vi "参数设置.vi"() -> ()   [LabVIEW 2018]
uses:
  globalMessage.vi
panel:
  in  "能量计量程":enum16{"200uJ", "20uJ", "2uJ", "200nJ"}(ring)
  in  "能量计通道":enum16{"Channel 1", "Channel 2"}(ring)=enum."Channel 2"
  in  "功率计通道":enum16{"Channel 1", "Channel 2"}(ring)
  in  "测量表头IP":string="192.168.129.77"
  in  "曝光时间 2":u64
  in  "模拟增益 2":u64
  in  "相机IP 2":string="192.168.1.10"
  in  "曝光时间":u64
  in  "模拟增益":u64
  in  "相机IP":string="192.168.1.10"
  in  "触发电压":u64(ring)=200 items=["200mv"=200, "20mv"=20, "2mv"=2]
  in  "时间范围":u64(ring)=100000 items=["100ms"=1000000000, "10ms"=100000000, "1ms"=10000000, "100us"=1000000, "10us"=100000, "1us"=10000, "100ns"=1000, "10ns"=100, "1ns"=10, "100ps"=1]
  in  "电压范围":u64(ring)=10 items=["1 V"=1000000, "100mv"=100000, "10mv"=10000, "1mv"=1000, "100uv"=100, "10uv"=10]
  in  "示波器通道":T1(ring)
  in  "工作波长（nm）":u32=400 min=400 max=1100
  in  "编号":string
  in  "激光器型号":string
  in  "确定":bool
  out "提示":string
  in  "error in (no error)":errorcluster
  # "通用参数"
  # "近场相机\n参数"
  # "远场相机\n参数"
  # "功率/能量计\n参数"
  # "示波器\n参数"
  # "偏振测量仪\n参数"
  # "光谱仪\n参数"
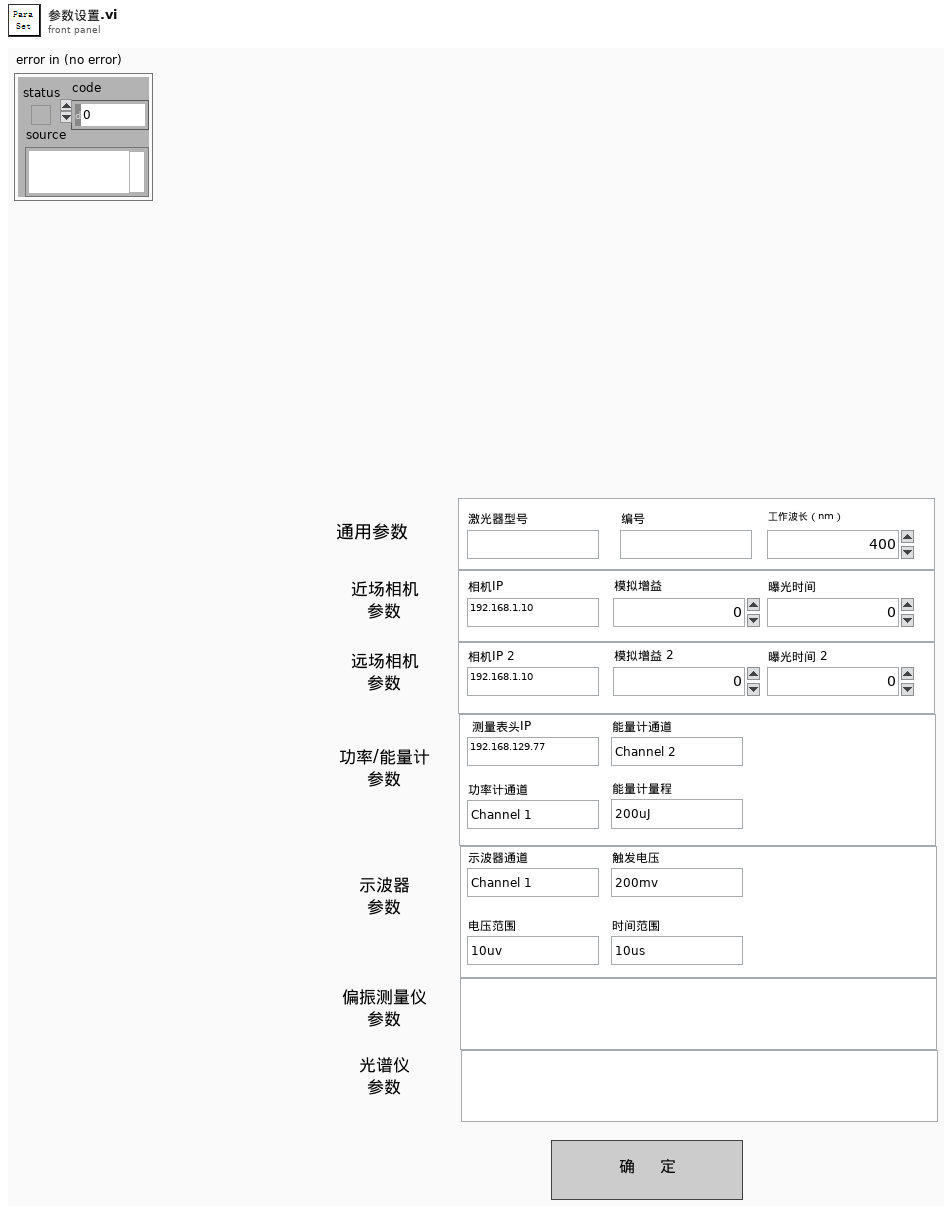
[diagram p1: front panel]
types:
  T1 = enum16{"Channel 1", "Channel 2", "Channel 3", "Channel 4"}
  T2 = typedef "Image Type" = u32
  T3 = typedef "IMAQ Image.ctl" = refnum<image>
  T4 = cluster{"激光器型号":string, "X":dbl, "Y":dbl, "Z":dbl, "Rotate":dbl, "Pitching":dbl}
  T5 = cluster{"示波器":cluster{"Channel (0:Channel 1)":enum16{"Channel 1", "Channel 2", "Channel 3", "Channel 4"}, "电压范围":dbl, "触发电压":dbl, "时间范围":dbl, " 示波器VISA":refnum<visa-resource-name>}, "光谱仪":cluster{"Channel (0:Channel 1)":enum16{"Channel 1", "Channel 2", "Channel 3", "Channel 4"}, "电压范围":u64, "触发电压":u64, "时间范围":u64}, " 近场相机":cluster{"曝光时间":i32, "模拟增益":i32, "控制套接字":i32, "IP 地址":string, " 采集套接字":i32, "  版本号":i32, "ImageData":T3, "  增益最大":i32, "  增益最小":i32, " 曝光最大":i32, " 曝光最小":i32, " 帧速":i32, " 同步切换":i32, "  曝光缩放":i32}, " 偏振仪":cluster{"电压范围":u64, "触发电压":u64, "时间范围":u64, "波长范围":enum16{"可见光 400-700nm", "近红外 700-1100nm"}}, " 功率计":cluster{"通道":enum16{"Channel 1", "Channel 2"}, "工作波长":u32, "单位":u64, "时间范围":u64, "IP地址":string, "端口":u32}, "能量计":cluster{"通道":enum16{"Channel 1", "Channel 2"}, "工作波长":u32, "单位":u64, "时间范围":u64, "IP地址":string, "端口":u32, "能量计量程":enum16{"200uJ", "20uJ", "2uJ", "200nJ"}}, "电机":cluster{"Channel (0:Channel 1)":enum16{"Channel 1", "Channel 2", "Channel 3", "Channel 4"}, "电压范围":u64, "触发电压":u64, "时间范围":u64}}
  T6 = cluster{"通道":enum16{"Channel 1", "Channel 2"}, "工作波长":u32, "单位":u64, "时间范围":u64, "IP地址":string, "端口":u32}
  T7 = cluster{"Channel (0:Channel 1)":enum16{"Channel 1", "Channel 2", "Channel 3", "Channel 4"}, "电压范围":dbl, "触发电压":dbl, "时间范围":dbl, " 示波器VISA":refnum<visa-resource-name>}
  T8 = cluster{"曝光时间":i32, "模拟增益":i32, "控制套接字":i32, "IP 地址":string, " 采集套接字":i32, "  版本号":i32, "ImageData":T3, "  增益最大":i32, "  增益最小":i32, " 曝光最大":i32, " 曝光最小":i32, " 帧速":i32, " 同步切换":i32, "  曝光缩放":i32}
  T9 = cluster{"通道":enum16{"Channel 1", "Channel 2"}, "工作波长":u32, "单位":u64, "时间范围":u64, "IP地址":string, "端口":u32, "能量计量程":enum16{"200uJ", "20uJ", "2uJ", "200nJ"}}
  T10 = cluster{"电压范围":u64, "触发电压":u64, "时间范围":u64, "波长范围":enum16{"可见光 400-700nm", "近红外 700-1100nm"}}
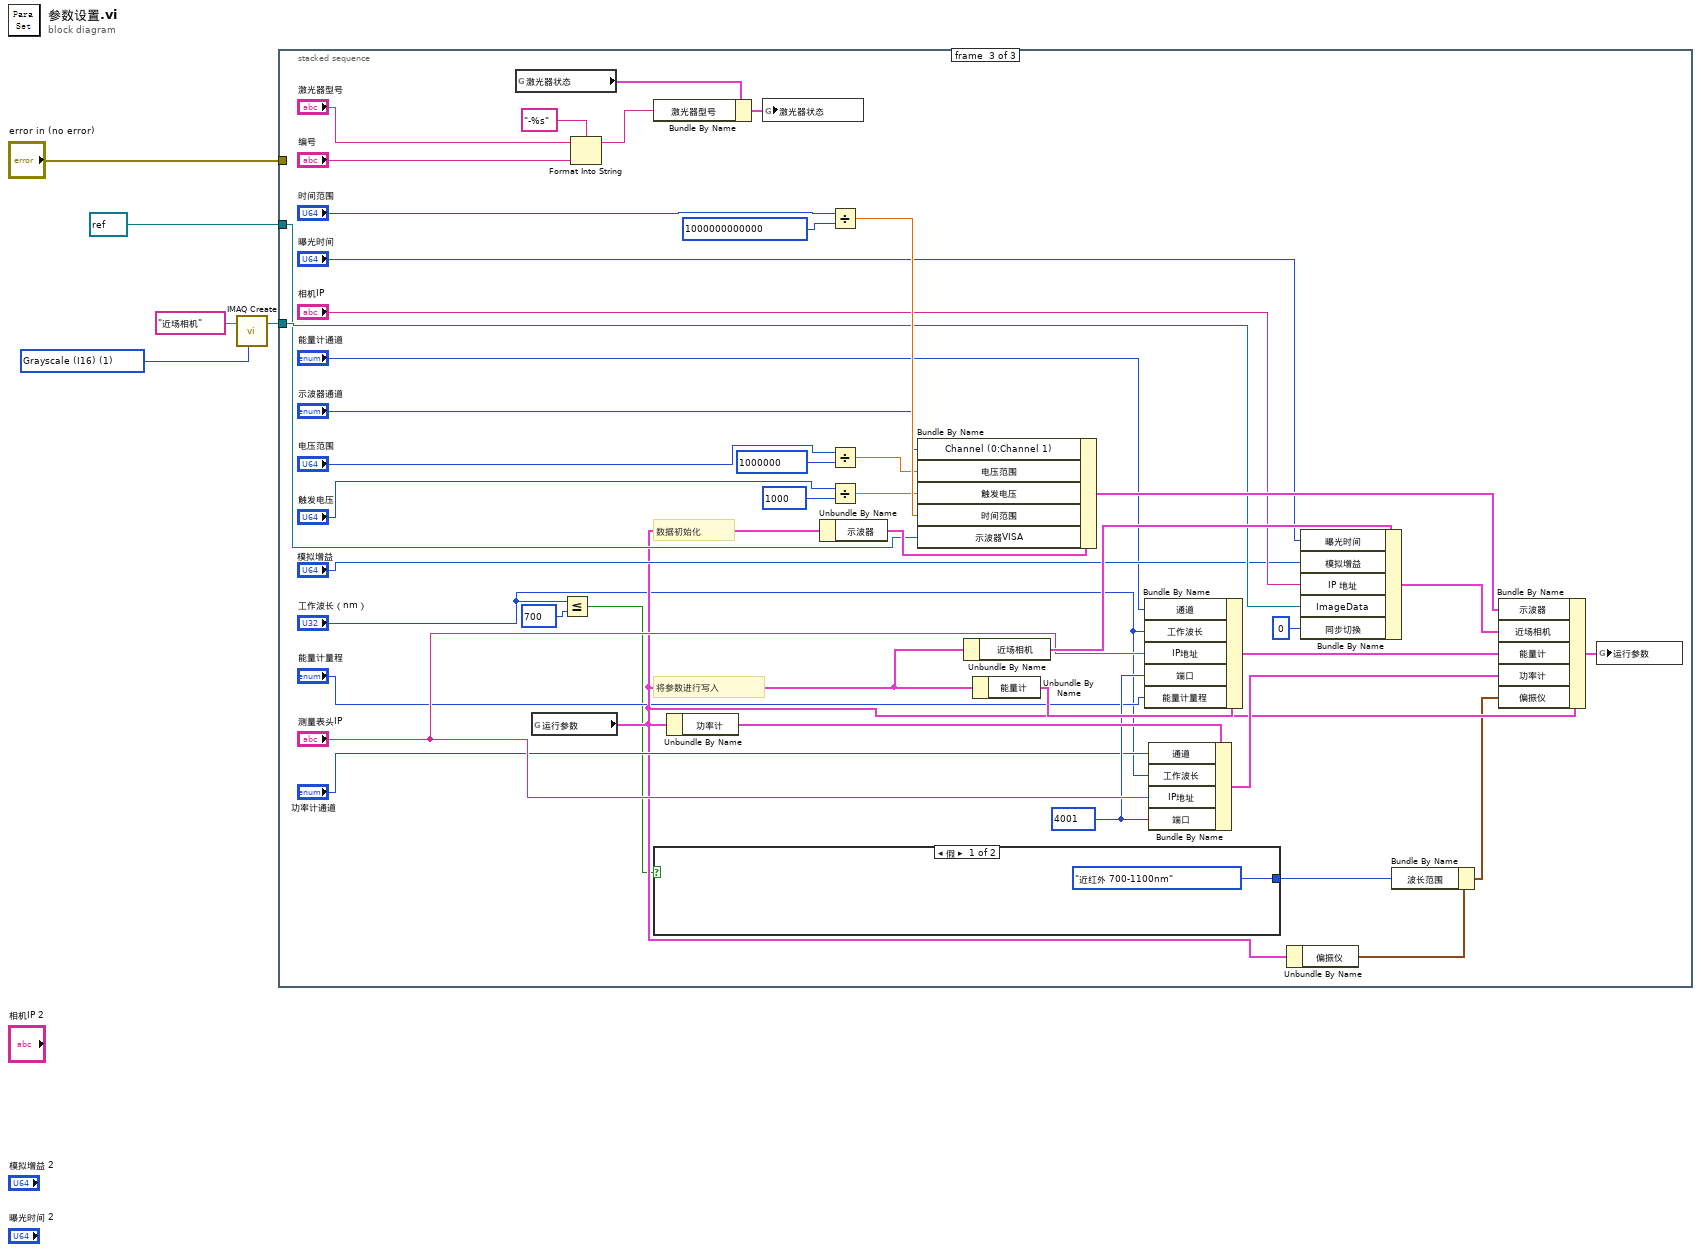
[diagram p0: block diagram]
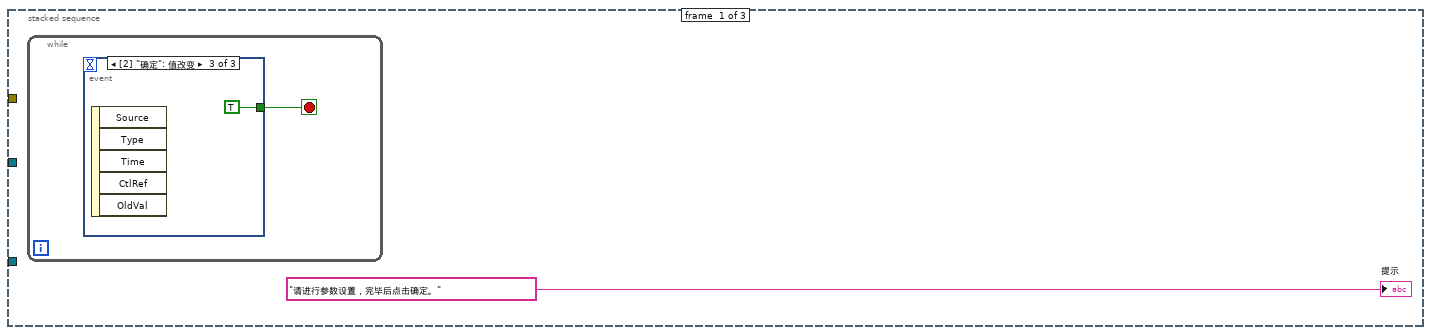
[diagram p2: hidden frame]
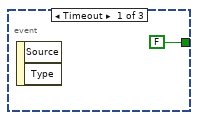
[diagram p3: hidden frame]
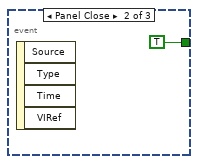
[diagram p4: hidden frame]
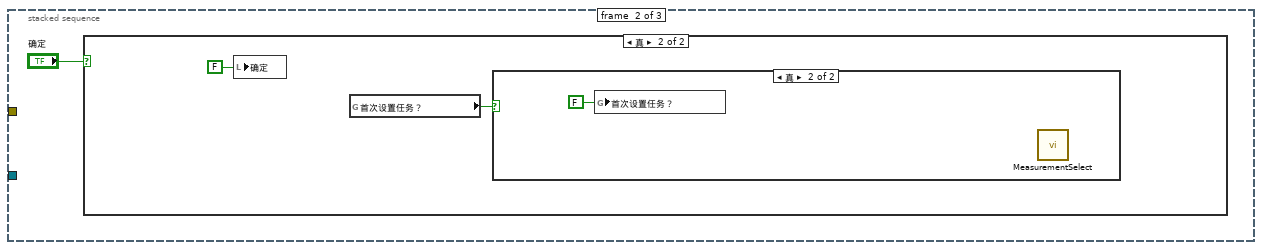
[diagram p5: hidden frame]
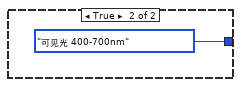
[diagram p8: hidden frame]
diagram:
  w2 = T2 1 items=["Grayscale (U8)", "Grayscale (I16)", "Grayscale (SGL)", "Complex (CSG)", "RGB (U32)", "HSL (U32)", "RGB (U64)", "Grayscale (U16)"] ("Image Type")
  n1 = call "IMAQ Create"("Image Name"="近场相机", "Image Type"=w2) -> ("New Image"=w3:T3)  [unwired: 3 in, 1 out]
  n2 = stacked-sequence {
    tunnel: "error in (no error)" -> [_ _ _]
    tunnel: w3 -> [_ _ w43]
    tunnel: refnum<visa-resource-name> refnum ("示波器VISA") -> [_ _ w37]
    frame #0 {
      n3 = while {
        stop <- w7 stop-if-true
        n4 = event shown="[2] \"确定\": 值改变" {
          selector: _ -> [_ _ _]
          dyn-events: _ -> [_ _ _]
          timeout: _ -> [_ _ _]
          tunnel: [FALSE TRUE TRUE] -> w7
          event Timeout {
            n5 = event-data() -> ()  [unwired: 1 in, 2 out]
          }
          event Panel Close {
            n6 = event-data() -> ()  [unwired: 1 in, 4 out]
          }
          event "确定": Value Change {
            n7 = event-data() -> ()  [unwired: 1 in, 5 out]
          }
        }
      }
      "提示" <- "请进行参数设置，完毕后点击确定。"
    }
    frame #1 {
      n8 = case shown="真" "确定" {
        frame False {
        }
        frame True {
          n9 = local write "确定"(FALSE ("确定")) -> ()
          n10 = global read "globalMessage.vi" "首次设置任务？"() -> (w13:bool)
          n11 = case shown="真" w13 {
            frame False {
            }
            frame True {
              n12 = global write "globalMessage.vi" "首次设置任务？"(FALSE ("首次设置任务？")) -> ()
              n13 = call "MeasurementSelect.vi"() -> ()  [unwired: 1 in, 1 out]
            }
          }
        }
      }
    }
    frame #2 {
      w31 = u32 4001
      # "将参数进行写入"
      # "数据初始化"
      n14 = global read "参数.vi" "激光器状态"() -> (w25:T4)
      n15 = global read "参数.vi" "运行参数"() -> (w28:T5)
      n16 = Less Or Equal?(x="工作波长（nm）", y=u32 700) -> (x <= y?=w15:bool)
      n17 = Format Into String(format string="-%s" ("格式字符串"), initial string="激光器型号", "编号") -> (resulting string=w20:string)  [unwired: 1 in, 1 out]
      n18 = Bundle By Name(cluster=w25, "激光器型号"=w20) -> (w24:T4)
      n19 = case shown="假" w15 {
        tunnel: [enum16{"可见光 400-700nm", "近红外 700-1100nm"}."近红外 700-1100nm" ("波长范围") enum16{"可见光 400-700nm", "近红外 700-1100nm"}."可见光 400-700nm" ("波长范围")] -> w16
        frame False {
        }
        frame True {
        }
      }
      n20 = Unbundle By Name(w28) -> ("功率计"=w36:T6)
      n21 = global write "参数.vi" "激光器状态"(w24) -> ()
      n22 = Unbundle By Name(w28) -> ("示波器"=w45:T7)
      n23 = Divide(x="时间范围", y=u64 1000000000000) -> (x/y=w51:dbl)
      n24 = Divide(x="电压范围", y=u64 1000000) -> (x/y=w49:dbl)
      n25 = Divide(x="触发电压", y=u64 1000) -> (x/y=w50:dbl)
      n26 = Bundle By Name(cluster=w45, "Channel (0:Channel 1)"="示波器通道", "电压范围"=w49, "触发电压"=w50, "时间范围"=w51, "示波器VISA"=w37) -> (w48:T7)
      n27 = Unbundle By Name(w28) -> ("近场相机"=w44:T8)
      n28 = Unbundle By Name(w28) -> ("能量计"=w35:T9)
      n29 = Bundle By Name(cluster=w35, "通道"="能量计通道", "工作波长"="工作波长（nm）", "IP地址"="测量表头IP", "端口"=w31, "能量计量程"="能量计量程") -> (w33:T9)
      n30 = Bundle By Name(cluster=w36, "通道"="功率计通道", "工作波长"="工作波长（nm）", "IP地址"="测量表头IP", "端口"=w31) -> (w34:T6)
      n31 = Unbundle By Name(w28) -> ("偏振仪"=w27:T10)
      n32 = Bundle By Name(cluster=w44, "曝光时间"="曝光时间", "模拟增益"="模拟增益", "IP 地址"="相机IP", "ImageData"=w43, "同步切换"=0) -> (w39:T8)
      n33 = Bundle By Name(cluster=w27, "波长范围"=w16) -> (w26:T10)
      n34 = Bundle By Name(cluster=w28, "示波器"=w48, "近场相机"=w39, "能量计"=w33, "功率计"=w34, "偏振仪"=w26) -> (w47:T5)
      n35 = global write "参数.vi" "运行参数"(w47) -> ()
    }
  }
